vi "mxwScript_Cmnd2Str_chainConnections.vi"(8 "error in (no error)":errorcluster, 11 "data":variant) -> (0 "error out":errorcluster, 3 "outputString":string)   [LabVIEW 2020]
uses:
  codeGenAPISupport.llb/cgAPI_mxwScript_Wire_ChainConnectionData.ctl
  codeGenAPISupport.llb/cgAPI_mxwScript_Wire_ChnCnnctStartEndData.ctl
  codeGenAPISupport.llb/cgAPI_mxwScript_ConnPaneArea.ctl
  codeGenAPISupport.llb/cgAPI_mxwScript_ConnPaneConnectionType.ctl
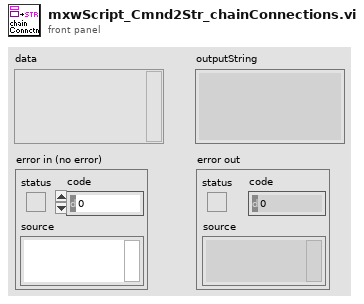
[diagram p1: front panel]
types:
  T1 = typedef "cgAPI_mxwScript_Wire_ChainConnectionData.ctl" = cluster{"source pattern":string, "sink pattern":string, "diagram ID":string, "internal?":bool, "connect first":T2, "connect last":T2}
  T2 = typedef "cgAPI_mxwScript_Wire_ChnCnnctStartEndData.ctl" = cluster{"connect?":bool, "final label":string, "use index?":bool, "connPaneIndex":i32, "area":T3, "connection type":T4}
  T3 = typedef "cgAPI_mxwScript_ConnPaneArea.ctl" = enum16{"TopLeft", "Top", "TopRight", "Right", "BottomRight", "Bottom", "BottomLeft", "Left"}
  T4 = typedef "cgAPI_mxwScript_ConnPaneConnectionType.ctl" = enum16{"Invalid Wire Rule", "Required", "Recommended", "Optional", "Dynamic Dispatch"}
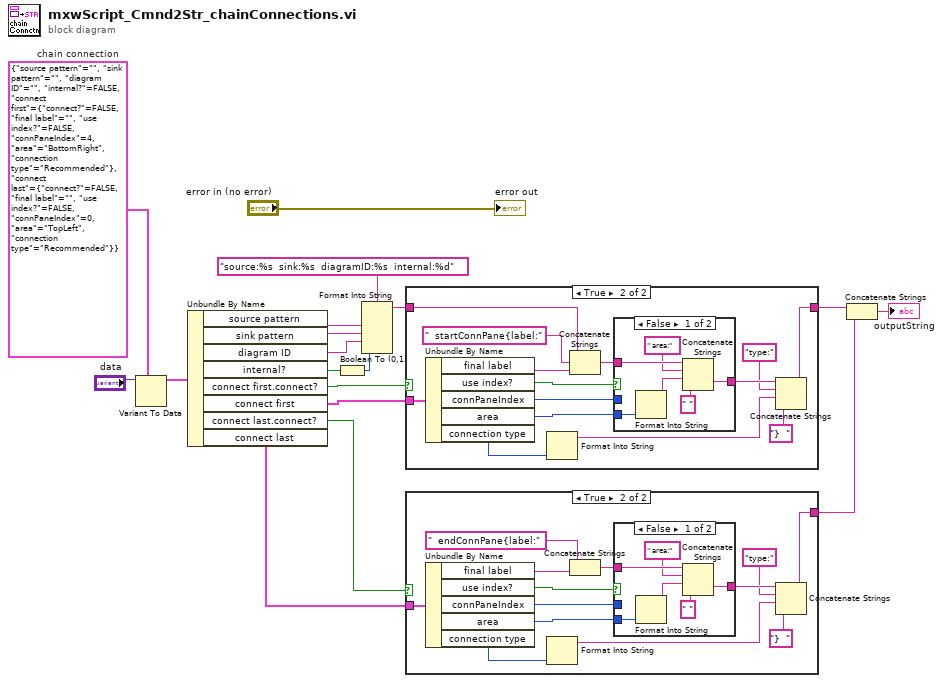
[diagram p0: block diagram]
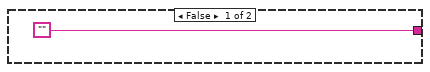
[diagram p2: hidden frame]
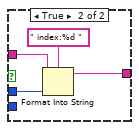
[diagram p3: hidden frame]
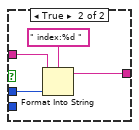
[diagram p5: hidden frame]
diagram:
  w14 = T1 {"source pattern"="", "sink pattern"="", "diagram ID"="", "internal?"=FALSE, "connect first"={"connect?"=FALSE, "final label"="", "use index?"=FALSE, "connPaneIndex"=4, "area"=enum."BottomRight", "connection type"=enum."Recommended"}, "connect last"={"connect?"=FALSE, "final label"="", "use index?"=FALSE, "connPaneIndex"=0, "area"=enum."TopLeft", "connection type"=enum."Recommended"}}  # chain connection
  n1 = Variant To Data(type=w14, Variant="data") -> (data=w17:T1)  [unwired: 1 in, 1 out]
  n2 = Unbundle By Name(w17) -> ("source pattern"=w12:string, "sink pattern"=w9:string, "diagram ID"=w10:string, "internal?"=w13:bool, "connect first.connect?"=w8:bool, "connect first"=w7:T2, "connect last.connect?"=w5:bool, "connect last"=w4:T2)
  n3 = Boolean To (0,1)(Boolean=w13) -> (0, 1=w11:i16)
  n4 = Format Into String(format string="source:%s  sink:%s  diagramID:%s  internal:%d", w12, w9, w10, w11) -> (resulting string=w6:string)  [unwired: 2 in, 1 out]
  n5 = case shown="True" w8 {
    tunnel: w7 -> [_ w33]
    tunnel: w6 -> [w19 w32]
    tunnel: [w19 w23] -> w3
    frame False {
    }
    frame True {
      n6 = Unbundle By Name(w33) -> ("final label"=w30:string, "use index?"=w28:bool, "connPaneIndex"=w27:i32, "area"=w26:T3, "connection type"=w29:T4)
      n7 = Format Into String(w29) -> (resulting string=w20:string)  [unwired: 3 in, 1 out]
      n8 = Concatenate Strings(w32, "  startConnPane{label:" ("string"), w30) -> (w25:string)
      n9 = case shown="False" w28 {
        tunnel: w27 -> [_ w41]
        tunnel: w26 -> [w39 _]
        tunnel: w25 -> [w38 w43]
        tunnel: [w34 w40] -> w24
        frame False {
          n10 = Format Into String(w39) -> (resulting string=w37:string)  [unwired: 3 in, 1 out]
          n11 = Concatenate Strings(w38, " area:" ("format string"), w37, " " ("string")) -> (w34:string)
        }
        frame True {
          n12 = Format Into String(format string=" index:%d ", initial string=w43, w41) -> (resulting string=w40:string)  [unwired: 1 in, 1 out]
        }
      }
      n13 = Concatenate Strings(w24, "type:" ("format string"), w20, "}  " ("string")) -> (w23:string)
    }
  }
  n14 = case shown="True" w5 {
    tunnel: w4 -> [_ w57]
    tunnel: ["" w48] -> w2
    frame False {
    }
    frame True {
      n15 = Unbundle By Name(w57) -> ("final label"=w55:string, "use index?"=w53:bool, "connPaneIndex"=w52:i32, "area"=w51:T3, "connection type"=w54:T4)
      n16 = Format Into String(w54) -> (resulting string=w45:string)  [unwired: 3 in, 1 out]
      n17 = Concatenate Strings("  endConnPane{label:" ("string"), w55) -> (w50:string)
      n18 = case shown="False" w53 {
        tunnel: w52 -> [_ w65]
        tunnel: w51 -> [w63 _]
        tunnel: w50 -> [w62 w67]
        tunnel: [w58 w64] -> w49
        frame False {
          n19 = Format Into String(w63) -> (resulting string=w61:string)  [unwired: 3 in, 1 out]
          n20 = Concatenate Strings(w62, " area:" ("format string"), w61, " " ("string")) -> (w58:string)
        }
        frame True {
          n21 = Format Into String(format string=" index:%d ", initial string=w67, w65) -> (resulting string=w64:string)  [unwired: 1 in, 1 out]
        }
      }
      n22 = Concatenate Strings(w49, "type:" ("format string"), w45, "}  " ("string")) -> (w48:string)
    }
  }
  n23 = Concatenate Strings(w3, w2) -> (→"outputString":string)
  "error out" <- "error in (no error)"
